vi "CheckForDeath.vi"(8 "error in (no error)":errorcluster, 11 "Snake in":refnum<class "SnakeGame.lvclass">) -> (0 "error out":errorcluster, 3 "Snake out":refnum<class "SnakeGame.lvclass">)   [LabVIEW 2019, in "RT_Game.lvlib" / "SnakeGame.lvclass"]
uses:
  SnakeGame.lvclass
  SnakeGame.lvclass/SnakeGame.ctl
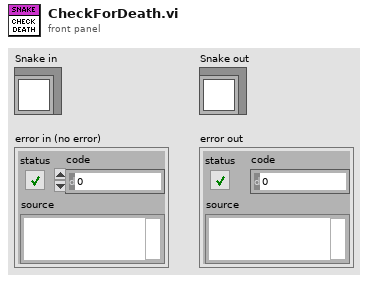
[diagram p1: front panel]
types:
  T1 = typedef "RT_Game.lvlib/SnakeGame.lvclass/CoordinateData.ctl" = cluster{"Coordinate":T2, "TileCode":string}
  T2 = typedef "RT_Game.lvlib/Game.lvclass/Coordinate.ctl" = cluster{"x":i16, "y":i16}
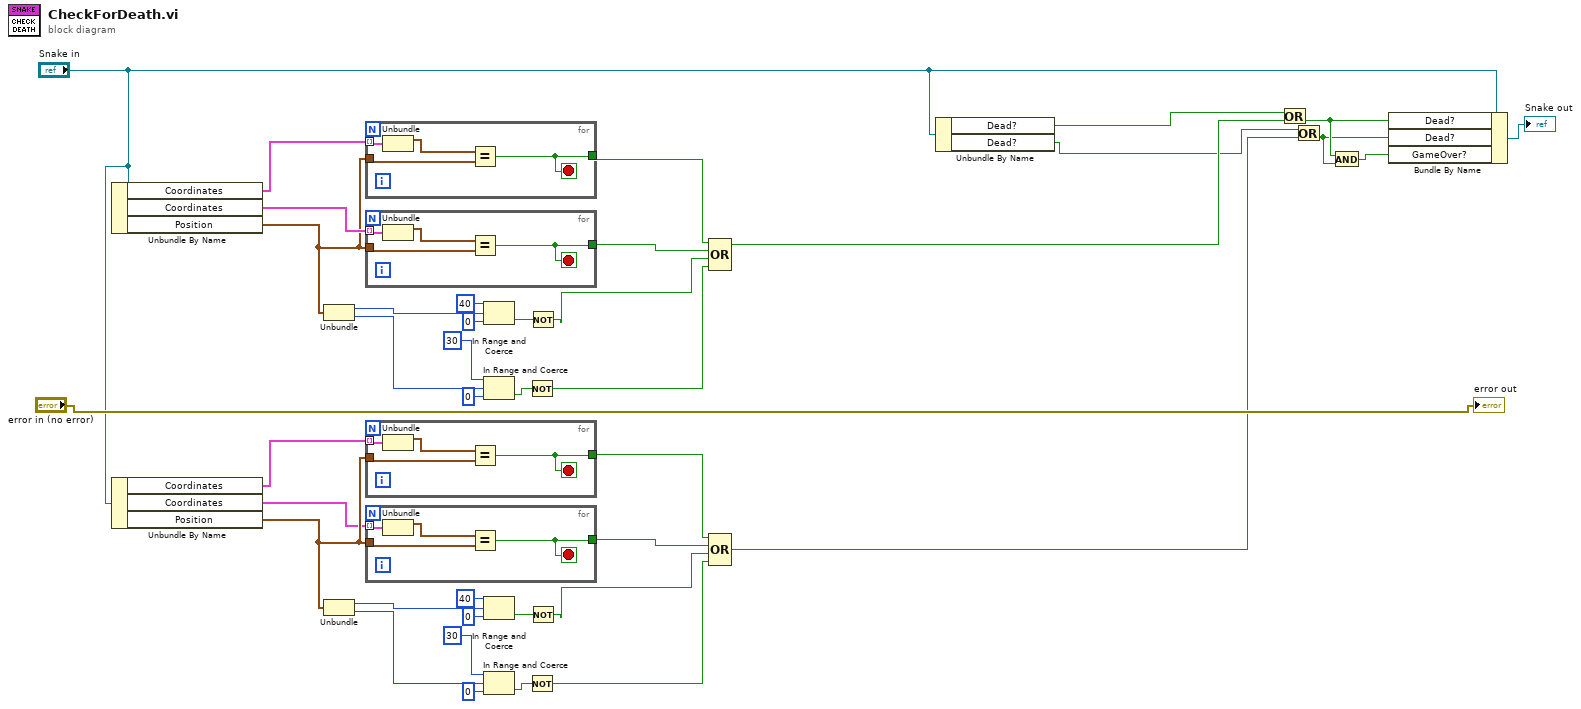
[diagram p0: block diagram]
diagram:
  n1 = Unbundle By Name("Snake in") -> ("Coordinates"=w26:T1[], "Coordinates"=w39:T1[], "Position"=w25:T2)
  n2 = Unbundle By Name("Snake in") -> ("Coordinates"=w21:T1[], "Coordinates"=w9:T1[], "Position"=w22:T2)
  n3 = Unbundle(w25) -> ("x"=w36:i16, "y"=w33:i16)
  n4 = Unbundle(w22) -> ("x"=w11:i16, "y"=w14:i16)
  n5 = for {
    tunnel: w26 -> [w43] mode=indexing
    tunnel: w25 -> [w44]
    tunnel: [w42] -> w24
    stop <- w42 stop-if-true
    n6 = Unbundle(w43) -> ("Coordinate"=w41:T2)  [unwired: 1 out]
    n7 = Equal?(x=w41, y=w44) -> (x = y?=w42:bool)
  }
  n8 = for {
    tunnel: w39 -> [w47] mode=indexing
    tunnel: w25 -> [w48]
    tunnel: [w46] -> w38
    stop <- w46 stop-if-true
    n9 = Unbundle(w47) -> ("Coordinate"=w45:T2)  [unwired: 1 out]
    n10 = Equal?(x=w45, y=w48) -> (x = y?=w46:bool)
  }
  n11 = for {
    tunnel: w21 -> [w51] mode=indexing
    tunnel: w22 -> [w52]
    tunnel: [w50] -> w23
    stop <- w50 stop-if-true
    n12 = Unbundle(w51) -> ("Coordinate"=w49:T2)  [unwired: 1 out]
    n13 = Equal?(x=w49, y=w52) -> (x = y?=w50:bool)
  }
  n14 = for {
    tunnel: w9 -> [w55] mode=indexing
    tunnel: w22 -> [w56]
    tunnel: [w54] -> w10
    stop <- w54 stop-if-true
    n15 = Unbundle(w55) -> ("Coordinate"=w53:T2)  [unwired: 1 out]
    n16 = Equal?(x=w53, y=w56) -> (x = y?=w54:bool)
  }
  n17 = In Range and Coerce(upper limit=i8 40, x=w36, lower limit=i8 0) -> (In Range?=w30:bool)  [unwired: 1 out]
  n18 = In Range and Coerce(upper limit=i8 30, x=w33, lower limit=i8 0) -> (In Range?=w29:bool)  [unwired: 1 out]
  n19 = In Range and Coerce(upper limit=i8 40, x=w11, lower limit=i8 0) -> (In Range?=w17:bool)  [unwired: 1 out]
  n20 = In Range and Coerce(upper limit=i8 30, x=w14, lower limit=i8 0) -> (In Range?=w18:bool)  [unwired: 1 out]
  n21 = Not(x=w29) -> (.not. x?=w27:bool)
  n22 = Not(x=w18) -> (.not. x?=w20:bool)
  n23 = Not(x=w30) -> (.not. x?=w28:bool)
  n24 = Not(x=w17) -> (.not. x?=w19:bool)
  n25 = Compound Arithmetic op=OR(w24, w38, w28, w27) -> (w37:bool)
  n26 = Compound Arithmetic op=OR(w23, w10, w19, w20) -> (w8:bool)
  n27 = Unbundle By Name("Snake in") -> ("Dead?"=w7:bool, "Dead?"=w6:bool)
  n28 = Or(x=w7, y=w37) -> (x .or. y?=w3:bool)
  n29 = Or(x=w6, y=w8) -> (x .or. y?=w2:bool)
  n30 = And(x=w3, y=w2) -> (x .and. y?=w1:bool)
  n31 = Bundle By Name(cluster="Snake in", "Dead?"=w3, "Dead?"=w2, "GameOver?"=w1) -> (→"Snake out":refnum<class "SnakeGame.lvclass">)
  "error out" <- "error in (no error)"
